vi "Solve1.vi"(8 "Error In":errorcluster, 11 "object in":refnum<class "2021_3.lvclass">) -> (0 "Error Out":errorcluster, 2 "Result":u64, 3 "object out":refnum<class "2021_3.lvclass">)   [LabVIEW 2020, in "2021_3.lvclass"]
uses:
  2021_3.lvclass
  2021_3.lvclass/2021_3.ctl
  6b7c88a8-8a6b-45f1-a591-125f7a5b4b0b.vi
  9b7eb7cf-65b9-4f49-bb16-e1a2974b5216.vi
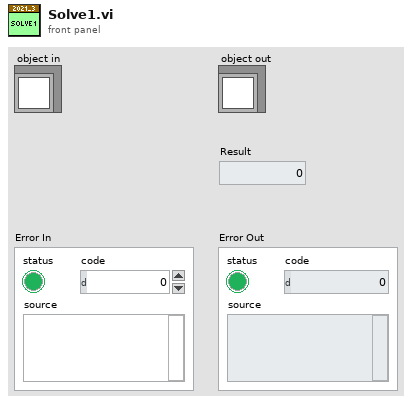
[diagram p1: front panel]
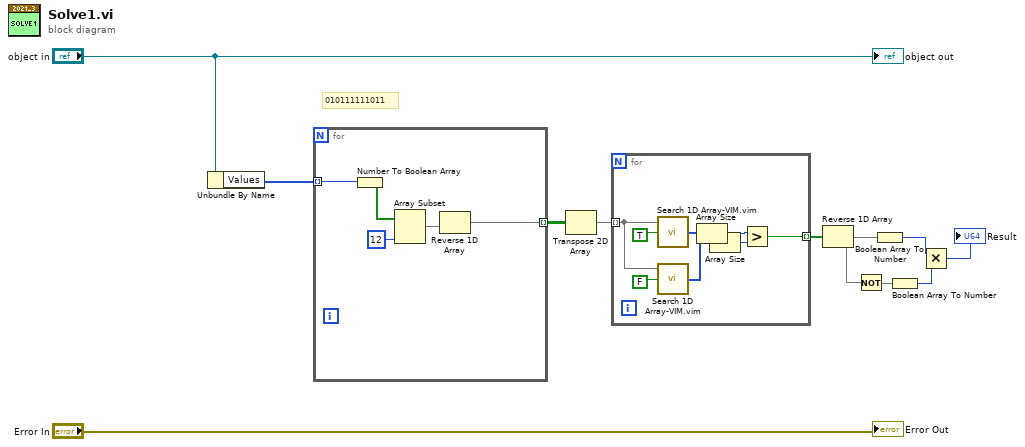
[diagram p0: block diagram]
diagram:
  # "010111111011"
  n1 = Unbundle By Name("object in") -> ("Values"=w9:u32[])
  n2 = for {
    tunnel: w9 -> [w16] mode=indexing
    tunnel: [w12] -> w8 mode=indexing
    n3 = Number To Boolean Array(number=w16) -> (Boolean array=w15:bool[])
    n4 = Array Subset(array=w15, length=12) -> (w13:bool[])  [unwired: 1 in]
    n5 = Reverse 1D Array(array=w13) -> (reversed array=w12:bool[])
  }
  n6 = Transpose 2D Array(2D array=w8) -> (transposed array=w7:bool[][])
  n7 = for {
    tunnel: w7 -> [w23] mode=indexing
    tunnel: [w17] -> w6 mode=indexing
    n8 = call "Search 1D Array-VIM.vim"("Array"=w23, "Element Data"=TRUE) -> ("Indices of Elements"=w21:i32[])  [unwired: 7 in]
    n9 = call "Search 1D Array-VIM.vim"("Array"=w23, "Element Data"=FALSE) -> ("Indices of Elements"=w20:i32[])  [unwired: 7 in]
    n10 = Array Size(array=w21) -> (size(s)=w19:i32)
    n11 = Array Size(array=w20) -> (size(s)=w18:i32)
    n12 = Greater?(x=w19, y=w18) -> (0:w17:bool)
  }
  n13 = Reverse 1D Array(array=w6) -> (reversed array=w5:bool[])
  n14 = Not(x=w5) -> (.not. x?=w4:bool[])
  n15 = Boolean Array To Number(Boolean array=w5) -> (number=w3:u32)
  n16 = Boolean Array To Number(Boolean array=w4) -> (number=w2:u32)
  n17 = Multiply(x=w3, y=w2) -> (x*y=→"Result":u32)
  "Error Out" <- "Error In"
  "object out" <- "object in"
